vi "בדיקת מתח שחרור של סליל פיקוד ללא עומס Mod.vi"(7 "resultUserPrompt":bool=TRUE, 8 "error":errorcluster, 9 "זמן סגירה מינימלי":dbl=1.5 format="%#_13g", 10 "שם הממסר":string="0410-24534 15A ממסר", 11 "Path for Log":path) -> (0 "error out":errorcluster, 1 "מצב ממסר פתוח/סגור":bool, 2 "מתח פתיחת הממסר":dbl format="%.4f", 3 "מתח מוצא מהספק":dbl format="%.4f")   [LabVIEW 2014]
uses:
  <vilib>/DAQmx/create/channels.llb/DAQmx Create Channel (DO-Digital Output).vi
  <vilib>/DAQmx/write.llb/DAQmx Write (Digital Bool 1Line 1Point).vi
panel:
  out "progress":dbl(slide) scale=0.0..11.0
  out "error IO DMM":errorcluster
  in  "Stop Button":bool
  # "Right-Click to\nexplain error"
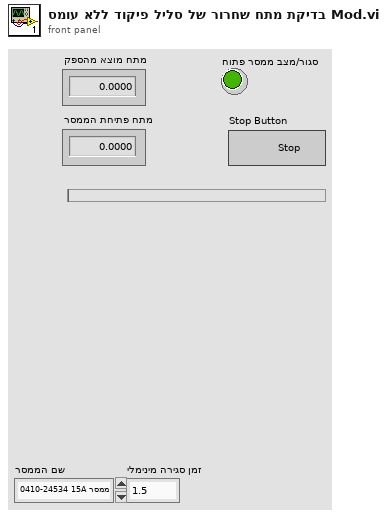
[diagram p1: front panel]
types:
  T1 = enum32{"Invalid", "Standard", "Closed", "Hidden", "Minimized", "Maximized"}
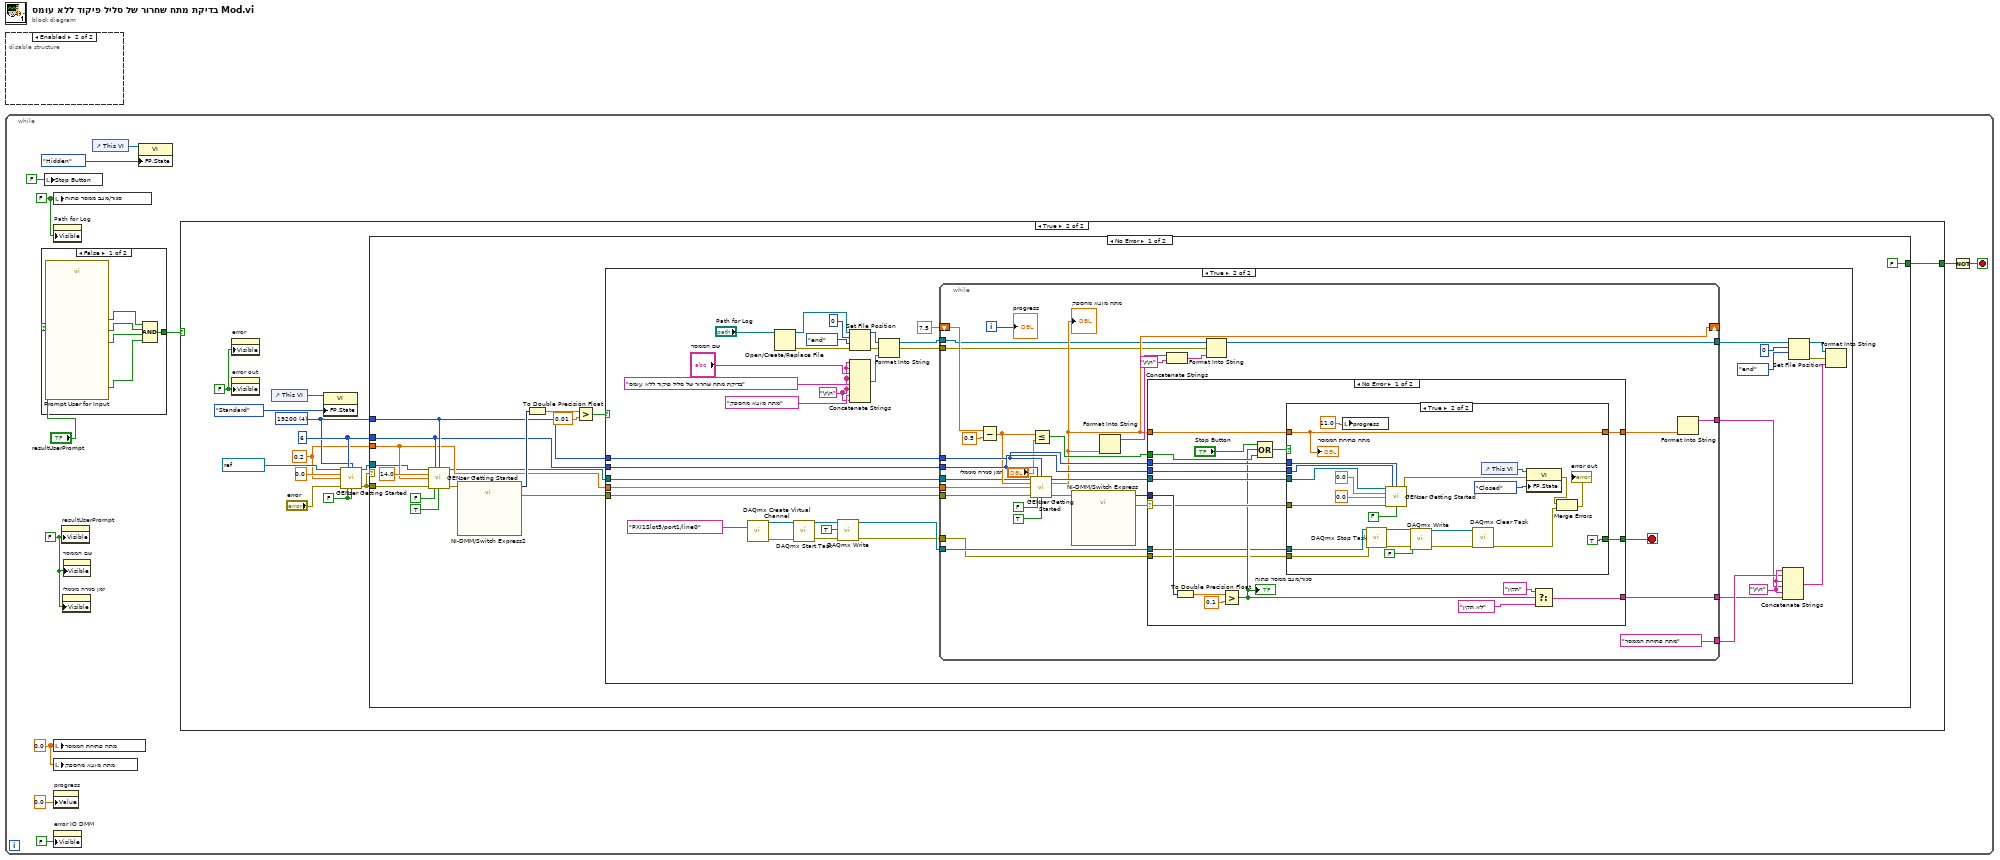
[diagram p0: block diagram]
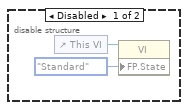
[diagram p2: hidden frame]
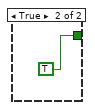
[diagram p3: hidden frame]
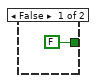
[diagram p4: hidden frame]
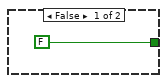
[diagram p6: hidden frame]
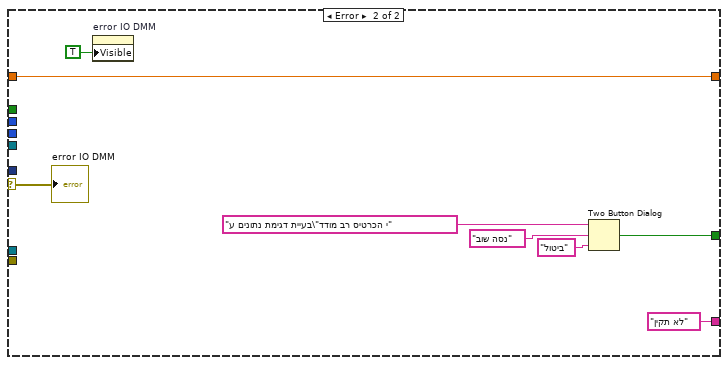
[diagram p7: hidden frame]
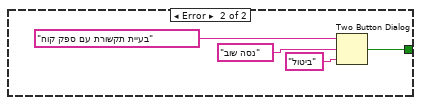
[diagram p8: hidden frame]
diagram:
  n1 = disable-structure shown="Enabled" {
    frame Disabled {
      n2 = control-ref of="This VI"() -> (w1:refnum<vi>)
      n3 = property class="VI"(reference=w1, "FP.State"=T1."Standard" ("Front Panel Window:State")) -> ()  [unwired: 1 in, 2 out]
    }
    frame Enabled {
    }
  }
  n4 = while {
    stop <- w14 stop-if-true
    w3 = FALSE ("Visible")
    w6 = FALSE ("מגע סגור")
    w9 = 0.0 ("signals out")
    n5 = case shown="False" "resultUserPrompt" {
      tunnel: [w19 TRUE] -> w4
      frame False {
        n6 = call "Prompt User for Input"() -> ("הדקי הרב מודד"=w15:bool, "מגע שלילי"=w16:bool, "מגע חיובי"=w17:bool, "OK"=w18:bool)  [unwired: 15 in, 1 out]
        n7 = Compound Arithmetic op=AND(w18, w17, w16, w15) -> (w19:bool)
      }
      frame True {
      }
    }
    n8 = local write "Stop Button"(FALSE ("Reset (T)")) -> ()
    n9 = local write "מצב ממסר פתוח/סגור"(w6) -> ()
    n10 = property on="Path for Log" class="Path"("Visible"=w6) -> ()  [unwired: 2 in, 2 out]
    n11 = local write "מתח פתיחת הממסר"(w9) -> ()
    n12 = local write "מתח מוצא מהספק"(w9) -> ()
    n13 = property on="progress" class="Slide (strict)"("Value"=0.0 ("progress")) -> ()  [unwired: 2 in, 2 out]
    n14 = property on="error IO DMM" class="Clust (strict)"("Visible"=FALSE) -> ()  [unwired: 2 in, 2 out]
    n15 = property on="resultUserPrompt" class="Bool (strict)"("Visible"=w3) -> ()  [unwired: 2 in, 2 out]
    n16 = property on="זמן סגירה מינימלי" class="DigNum (strict)"("Visible"=w3) -> ()  [unwired: 2 in, 2 out]
    n17 = property on="שם הממסר" class="Str"("Visible"=w3) -> ()  [unwired: 2 in, 2 out]
    n18 = control-ref of="This VI"() -> (w8:refnum<vi>)
    n19 = property class="VI"(reference=w8, "FP.State"=T1."Hidden" ("Front Panel Window:State")) -> ()  [unwired: 1 in, 2 out]
    n20 = case shown="True" w4 {
      tunnel: [FALSE ("T button?") w26] -> w13
      frame False {
      }
      frame True {
        w24 = FALSE ("Visible")
        w25 = FALSE ("Output On (T)")
        w30 = u16 4 items=["1200", "2400", "4800", "9600", "19200"] ("BAUD")
        w31 = i16 6 ("GEN Addr")
        w27 = 0.2 ("Current Limit")
        n21 = property on="error" class="Clust (strict)"("Visible"=w24) -> ()  [unwired: 2 in, 2 out]
        n22 = property on="error out" class="Clust (strict)"("Visible"=w24) -> ()  [unwired: 2 in, 2 out]
        n23 = control-ref of="This VI"() -> (w22:refnum<vi>)
        n24 = property class="VI"(reference=w22, "FP.State"=T1."Standard" ("Front Panel Window:State")) -> ()  [unwired: 1 in, 2 out]
        n25 = call "GENser Getting Started.vi"("VISA"=refnum<visa-resource-name> "COM6", "GEN Addr"=w31, "BAUD"=w30, "Voltage Limit"=0.0, "Current Limit"=w27, "error"="error", "Reset (T)"=w25, "Output On (T)"=w25) -> ("VISA out"=w32:refnum<visa-resource-name>, "error out"=w33:errorcluster)  [unwired: 4 in, 2 out]
        n26 = case shown="No Error" w33 {
          tunnel: w33 -> [w42 _]
          tunnel: w32 -> [w38 _]
          tunnel: w31 -> [w40 _]
          tunnel: w30 -> [w41 _]
          tunnel: w27 -> [w39 _]
          tunnel: [FALSE w171] -> w26
          frame No Error {
            n27 = call "GENser Getting Started.vi"("VISA"=w38, "GEN Addr"=w40, "BAUD"=w41, "Voltage Limit"=14.0, "Current Limit"=w39, "error"=w42, "Reset (T)"=FALSE, "Output On (T)"=TRUE) -> ("VISA out"=w37:refnum<visa-resource-name>, "error out"=w46:errorcluster)  [unwired: 4 in, 2 out]
            n28 = call "NI-DMM/Switch Express2"("error in"=w46) -> ("signals out"=w45:dynamicdata, "error out"=w43:errorcluster)  [unwired: 16 in, 1 out]
            n29 = To Double Precision Float(number=w45) -> (double precision float=w36:dbl)
            n30 = Greater?(x=w36, y=0.01) -> (0:w44:bool)
            n31 = case shown="True" w44 {
              tunnel: w43 -> [_ w88]
              tunnel: w40 -> [_ w87]
              tunnel: w41 -> [_ w86]
              tunnel: w39 -> [_ w85]
              tunnel: w37 -> [_ w83]
              frame False {
              }
              frame True {
                w59 = "\r\n"
                w82 = "\r\n"
                n32 = call-poly <vilib>:"DAQmx Create Virtual Channel.vi"("lines"=tag "PXI1Slot5/port1/line0") -> ("task out"=w57:refnum<k21>, "error out"=w58:errorcluster)  [unwired: 13 in]
                n33 = Open/Create/Replace File(file path (use dialog)="Path for Log") -> (refnum out=w70:refnum<file>, error out=w69:errorcluster)  [unwired: 5 in, 1 out]
                n34 = call <vilib>:"DAQmx Start Task.vi"("task/channels in"=w57, "error in"=w58) -> ("task out"=w55:refnum<k21>, "error out"=w54:errorcluster)  [unwired: 12 in]
                n35 = call-poly <vilib>:"DAQmx Write.vi"("task/channels in"=w55, "data"=TRUE, "error in"=w54) -> ("task out"=w52:refnum<k21>, "error out"=w51:errorcluster)  [unwired: 10 in, 1 out]
                n36 = Set File Position(offset (in bytes) (0)=i64 0, refnum=w70, from (0:start)=enum16{"start", "end", "current"}."end", error in=w69) -> (refnum out=w65:refnum<file>, error out=w60:errorcluster)
                n37 = Concatenate Strings(w59, w59, "שם הממסר", w59, "בדיקת מתח שחרור של סליל פיקוד ללא עומס", w59, "מתח מוצא מהספק", w59) -> (w68:string)
                n38 = Format Into String(initial string=w65, error in=w60, w68) -> (resulting string=w62:refnum<file>, error out=w61:errorcluster)  [unwired: 1 in]
                n39 = while {
                  tunnel: w88 -> [w119]
                  tunnel: w87 -> [w111]
                  tunnel: w86 -> [w110]
                  tunnel: w85 -> [w117]
                  shift-right: [w93] -> _
                  shift-left: 7.5 ("y") -> [w115]
                  tunnel: w83 -> [w103]
                  tunnel: [w98] -> w77
                  tunnel: ["מתח פתיחת הממסר"] -> w76
                  tunnel: [w96] -> w75
                  tunnel: [w95] -> w74
                  tunnel: w62 -> [w92]
                  tunnel: w61 -> [w91]
                  tunnel: w52 -> [w90]
                  tunnel: w51 -> [w89]
                  i -> [w104]
                  stop <- w112 stop-if-true
                  n40 = Subtract(x=w115, y=0.5) -> (x-y=w107:dbl)
                  n41 = call "GENser Getting Started.vi"("VISA"=w103, "GEN Addr"=w111, "BAUD"=w110, "Voltage Limit"=w107, "Current Limit"=w117, "error"=w119, "Reset (T)"=FALSE, "Output On (T)"=TRUE) -> ("VISA out"=w109:refnum<visa-resource-name>, "Output Voltage"=w93:dbl, "error out"=w114:errorcluster)  [unwired: 4 in, 1 out]
                  "מתח מוצא מהספק" <- w93
                  n42 = Less Or Equal?(x=w107, y="זמן סגירה מינימלי") -> (x <= y?=w106:bool)
                  n43 = call "NI-DMM/Switch Express"("error in"=w114) -> ("signals out"=w113:dynamicdata, "error out"=w105:errorcluster)  [unwired: 16 in, 1 out]
                  n44 = Format Into String(w93) -> (resulting string=w100:string)  [unwired: 3 in, 1 out]
                  n45 = case shown="No Error" w105 {
                    selector: w105 -> [w129 w170]
                    tunnel: w113 -> [w138 _]
                    tunnel: [w135 w166] -> w112
                    tunnel: w111 -> [w134 _]
                    tunnel: w110 -> [w133 _]
                    tunnel: w109 -> [w132 _]
                    tunnel: w106 -> [w131 _]
                    tunnel: w93 -> [w130 w164]
                    tunnel: [w123 w164] -> w99
                    tunnel: [w122 "לא תקין"] -> w95
                    tunnel: w90 -> [w121 _]
                    tunnel: w89 -> [w120 _]
                    frame No Error {
                      n46 = To Double Precision Float(number=w138) -> (double precision float=w128:dbl)
                      n47 = Greater?(x=w128, y=0.1) -> (0:w124:bool)
                      "מצב ממסר פתוח/סגור" <- w124
                      n48 = Compound Arithmetic op=OR("Stop Button", w124, w131) -> (w137:bool)
                      n49 = case shown="True" w137 {
                        tunnel: [FALSE TRUE] -> w135
                        tunnel: w134 -> [_ w161]
                        tunnel: w133 -> [_ w160]
                        tunnel: w132 -> [_ w159]
                        tunnel: w129 -> [_ w156]
                        tunnel: w130 -> [_ w150]
                        tunnel: [_ w150] -> w123
                        tunnel: w121 -> [_ w144]
                        tunnel: w120 -> [_ w143]
                        frame False {
                        }
                        frame True {
                          n50 = local write "progress"(11.0 ("progress")) -> ()
                          n51 = call <vilib>:"DAQmx Stop Task.vi"("task/channels in"=w144, "error in"=w143) -> ("task out"=w149:refnum<k21>, "error out"=w148:errorcluster)  [unwired: 12 in]
                          n52 = call "GENser Getting Started.vi"("VISA"=w159, "GEN Addr"=w161, "BAUD"=w160, "Voltage Limit"=0.0, "Current Limit"=0.0, "error"=w156, "Output On (T)"=FALSE) -> ("error out"=w151:errorcluster)  [unwired: 5 in, 3 out]
                          n53 = call-poly <vilib>:"DAQmx Write.vi"("task/channels in"=w149, "data"=FALSE, "error in"=w148) -> ("task out"=w147:refnum<k21>, "error out"=w146:errorcluster)  [unwired: 10 in, 1 out]
                          n54 = call <vilib>:"DAQmx Clear Task.vi"("task in"=w147, "error in"=w146) -> ("error out"=w142:errorcluster)  [unwired: 13 in]
                          n55 = control-ref of="This VI"() -> (w152:refnum<vi>)
                          n56 = property class="VI"(reference=w152, error in=w151, "FP.State"=T1."Closed" ("Front Panel Window:State")) -> (error out=w141:errorcluster)  [unwired: 1 out]
                          n57 = Merge Errors(w141, w142) -> (→"error out":errorcluster)
                          "מתח פתיחת הממסר" <- w150
                        }
                      }
                      n58 = Select(t="תקין", s=w124, f="לא תקין") -> (s? t:f=w122:string)
                    }
                    frame Error {
                      n59 = property on="error IO DMM" class="Clust (strict)"("Visible"=TRUE) -> ()  [unwired: 2 in, 2 out]
                      n60 = Two Button Dialog(message="בעיית דגימת נתונים ע\"י הכרטיס רב מודד", 1:"ביטול" ("F button name (\"Cancel\")"), 2:"נסה שוב" ("T button name (\"OK\")")) -> (T button?=w166:bool)
                      "error IO DMM" <- w170
                    }
                  }
                  n61 = Concatenate Strings(w100, "\r\n") -> (w94:string)
                  n62 = Format Into String(initial string=w92, error in=w91, w94) -> (resulting string=w98:refnum<file>)  [unwired: 1 in, 1 out]
                  n63 = Format Into String(w99) -> (resulting string=w96:string)  [unwired: 3 in, 1 out]
                  "progress" <- w104
                }
                n64 = Concatenate Strings(w82, w76, w82, w75, w82, w74) -> (w73:string)
                n65 = Set File Position(offset (in bytes) (0)=i64 0, refnum=w77, from (0:start)=enum16{"start", "end", "current"}."end") -> (refnum out=w79:refnum<file>, error out=w78:errorcluster)  [unwired: 1 in]
                n66 = Format Into String(initial string=w79, error in=w78, w73) -> ()  [unwired: 1 in, 2 out]
              }
            }
          }
          frame Error {
            n67 = Two Button Dialog(message="בעיית תקשורת עם ספק קוח", 1:"ביטול" ("F button name (\"Cancel\")"), 2:"נסה שוב" ("T button name (\"OK\")")) -> (T button?=w171:bool)
          }
        }
      }
    }
    n68 = Not(x=w13) -> (.not. x?=w14:bool)
  }
